vi "Set First Val_LIN.vi"(6 "Payload LIN":u32[](array[numeric])=[0, 0, 0, 0, 0, 0, 0, 0] format="%x", 8 "error in":errorcluster, 9 "DLC LIN":u32, 10 "ID LIN":u32 format="%x", 11 "gRPC ID":T1) -> (0 "error out":errorcluster, 3 "gRPC ID out":T1)   [LabVIEW 2025, in "CAN-LIN Frame Generator UI.lvlib"]
uses:
  CAN-LIN Frame Generator UI.lvlib
  <vilib>/gRPC/LabVIEW gRPC Library/Shared/grpcId.ctl
  OOB gRPC Client/RPC Messages/hwval_GenericRequest.ctl
  OOB gRPC Client/OOB gRPC Client.lvlib
  <vilib>/gRPC/LabVIEW gRPC Library/grpc-lvsupport-release.lvlib
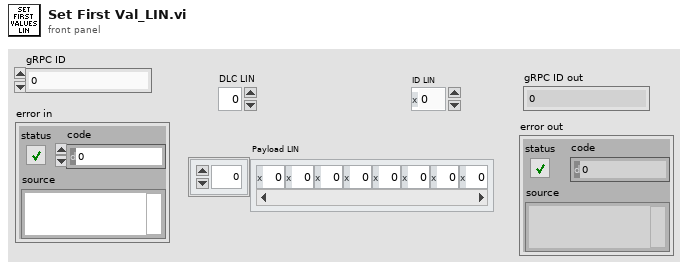
[diagram p1: front panel]
types:
  T1 = typedef "grpc-lvsupport-release.lvlib/grpcId.ctl" = u64
  T2 = typedef "OOB gRPC Client.lvlib/hwval_GenericRequest.ctl" = cluster{"Command":string, "Payload":u8[]}
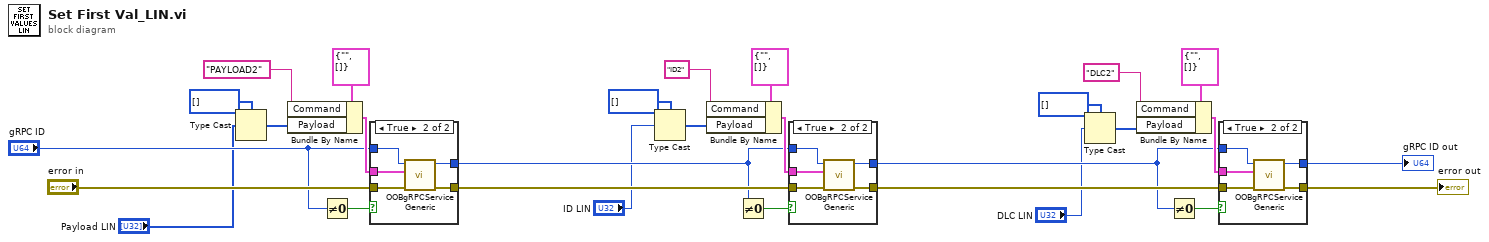
[diagram p0: block diagram]
diagram:
  n1 = Type Cast(type=u8[] [] ("Payload"), x="Payload LIN") -> (*(type *) &x=w26:u8[])
  n2 = Bundle By Name(cluster=T2 {"Command"="", "Payload"=[]} ("hwval_GenericRequest"), "Command"="PAYLOAD2", "Payload"=w26) -> (w25:T2)
  n3 = Not Equal To 0?(x="gRPC ID") -> (x != 0?=w24:bool)
  n4 = case shown="True" w24 {
    tunnel: [w30 w35] -> w7
    tunnel: [w31 w34] -> w8
    tunnel: "error in" -> [w31 w32]
    tunnel: w25 -> [_ w36]
    tunnel: "gRPC ID" -> [w30 w33]
    frame False {
    }
    frame True {
      n5 = call "OOBgRPCService Generic.vi"("error in"=w32, "Request Data"=w36, "gRPC ID"=w33) -> ("error out"=w34:errorcluster, "gRPC ID out"=w35:T1)  [unwired: 6 in, 1 out]
    }
  }
  n6 = Type Cast(type=u8[] [] ("Payload"), x="ID LIN") -> (*(type *) &x=w18:u8[])
  n7 = Bundle By Name(cluster=T2 {"Command"="", "Payload"=[]} ("hwval_GenericRequest"), "Command"="ID2", "Payload"=w18) -> (w19:T2)
  n8 = Not Equal To 0?(x=w7) -> (x != 0?=w20:bool)
  n9 = case shown="True" w20 {
    tunnel: [w37 w42] -> w5
    tunnel: [w38 w41] -> w6
    tunnel: w8 -> [w38 w39]
    tunnel: w19 -> [_ w43]
    tunnel: w7 -> [w37 w40]
    frame False {
    }
    frame True {
      n10 = call "OOBgRPCService Generic.vi"("error in"=w39, "Request Data"=w43, "gRPC ID"=w40) -> ("error out"=w41:errorcluster, "gRPC ID out"=w42:T1)  [unwired: 6 in, 1 out]
    }
  }
  n11 = Type Cast(type=u8[] [] ("Payload"), x="DLC LIN") -> (*(type *) &x=w11:u8[])
  n12 = Bundle By Name(cluster=T2 {"Command"="", "Payload"=[]} ("hwval_GenericRequest"), "Command"="DLC2", "Payload"=w11) -> (w10:T2)
  n13 = Not Equal To 0?(x=w5) -> (x != 0?=w9:bool)
  n14 = case shown="True" w9 {
    tunnel: [w44 w49] -> w4
    tunnel: [w45 w48] -> w3
    tunnel: w6 -> [w45 w46]
    tunnel: w10 -> [_ w50]
    tunnel: w5 -> [w44 w47]
    frame False {
    }
    frame True {
      n15 = call "OOBgRPCService Generic.vi"("error in"=w46, "Request Data"=w50, "gRPC ID"=w47) -> ("error out"=w48:errorcluster, "gRPC ID out"=w49:T1)  [unwired: 6 in, 1 out]
    }
  }
  "error out" <- w3
  "gRPC ID out" <- w4
